vi "Configure RemIO Module Core.vi"(8 "error in (no error)":errorcluster, 9 "module slot index":u8=1, 10 "Slave Ref In":refnum<k21>, 11 "RemIO Module in":refnum<class "RemIO Module.lvclass">) -> (0 "error out":errorcluster, 1 "negative confirmation":T1 {"additional error code" format="%.0x"; "error code" format="%.0x"}, 2 "Slave Ref Out":refnum<k21>, 3 "RemIO Module out":refnum<class "RemIO Module.lvclass">, 5 "SDO abort code":u32 format="%.0x")   [LabVIEW 2017, in "Modules.lvlib" / "RemIO Module.lvclass"]
uses:
  RemIO Module.lvclass
  <vilib>/indcomecat/Remote IO/typedefs/negative confirmation.ctl
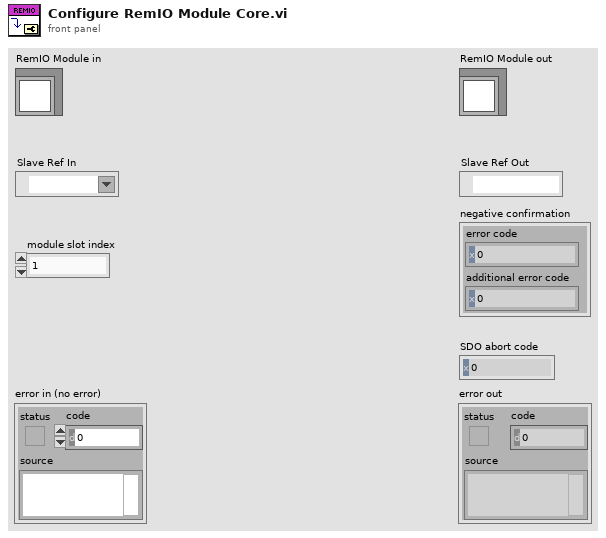
[diagram p1: front panel]
types:
  T1 = typedef "negative confirmation.ctl" = cluster{"error code":u16, "additional error code":u16}
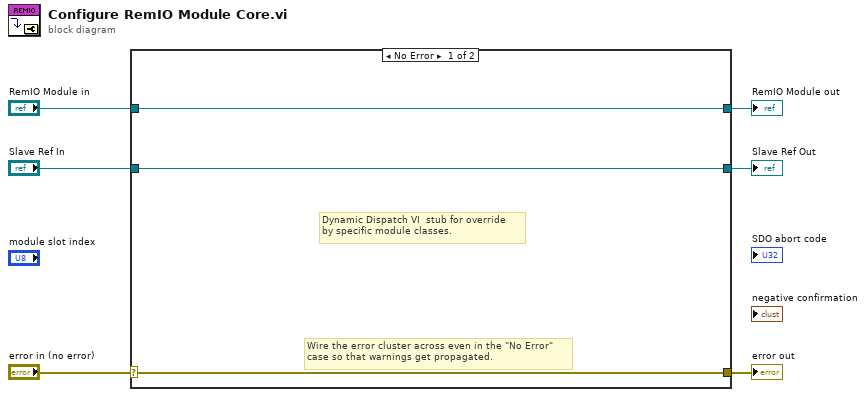
[diagram p0: block diagram]
diagram:
  n1 = case shown="No Error" "error in (no error)" {
    selector: "error in (no error)" -> [w8 w12]
    tunnel: [w8 w12] -> w5
    tunnel: [w9 w11] -> w3
    tunnel: "RemIO Module in" -> [w9 w11]
    tunnel: "Slave Ref In" -> [w7 w10]
    tunnel: [w7 w10] -> w1
    frame No Error {
      # "Dynamic Dispatch VI  stub for override\nby specific module classes."
      # "Wire the error cluster across even in the \"No Error\"\ncase so that warnings get propagated."
    }
    frame Error {
    }
  }
  "error out" <- w5
  "RemIO Module out" <- w3
  "Slave Ref Out" <- w1
